vi "차트와 그래프 차이 예제.vi"() -> ()   [LabVIEW 2025]
uses:
  <vilib>/numeric/Random Number (Range) U64.vi
  <vilib>/numeric/sub_Random U32.vi
panel:
  out "waveform":waveform(dbl)
  out "Waveform Graph":u64[](graph)
  out "Waveform Chart":u64(graph)
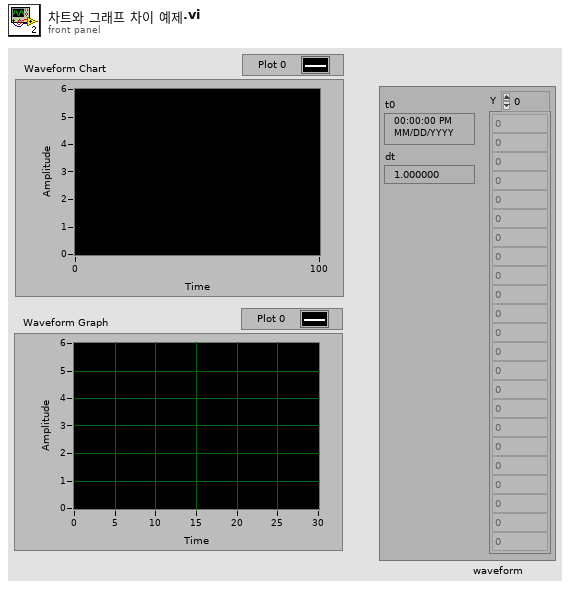
[diagram p1: front panel]
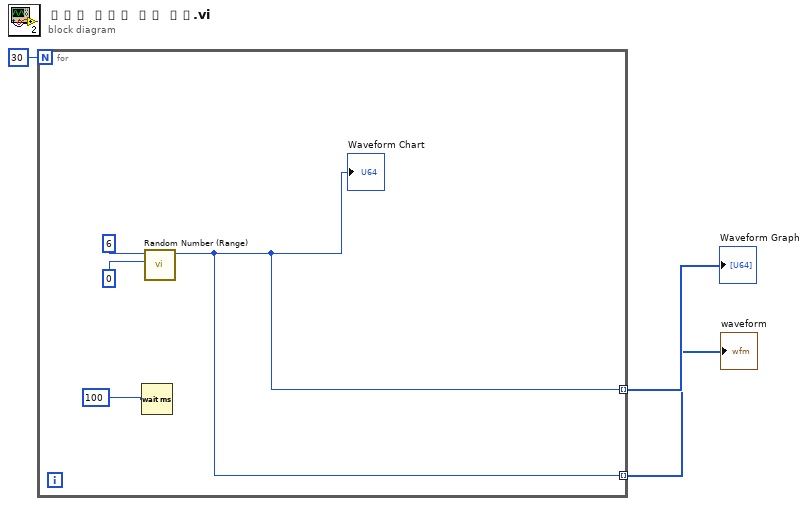
[diagram p0: block diagram]
diagram:
  n1 = for {
    N: 30 -> [_]
    tunnel: [w4] -> w2 mode=indexing
    tunnel: [w4] -> w1 mode=indexing
    n2 = Wait (ms)(milliseconds to wait=u32 100) -> ()  [unwired: 1 out]
    n3 = call-poly <vilib>:"Random Number (Range).vi"("lower bound (0)"=u64 0, "upper bound (100)"=u64 6) -> ("number"=w4:u64)  [unwired: 9 in]
    "Waveform Chart" <- w4
  }
  "Waveform Graph" <- w2
  "waveform" <- w1
